vi "Timer On Delay.vi"(8 "error in":errorcluster, 10 "preset time (ms)":i32=1000, 11 "input":bool) -> (0 "error out":errorcluster, 2 "elapsed time (ms)":i32, 3 "output":bool)   [LabVIEW 2012, in "毫秒定时器.lvlib"]
uses:
  <vilib>/ptbypt/NI_PtbyPt.lvlib
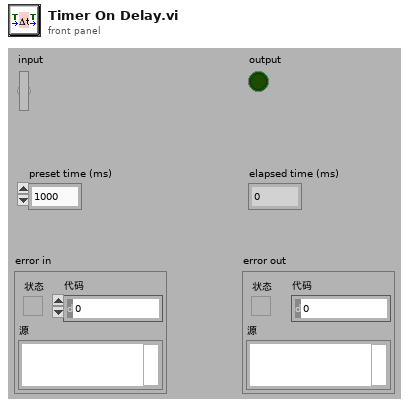
[diagram p1: front panel]
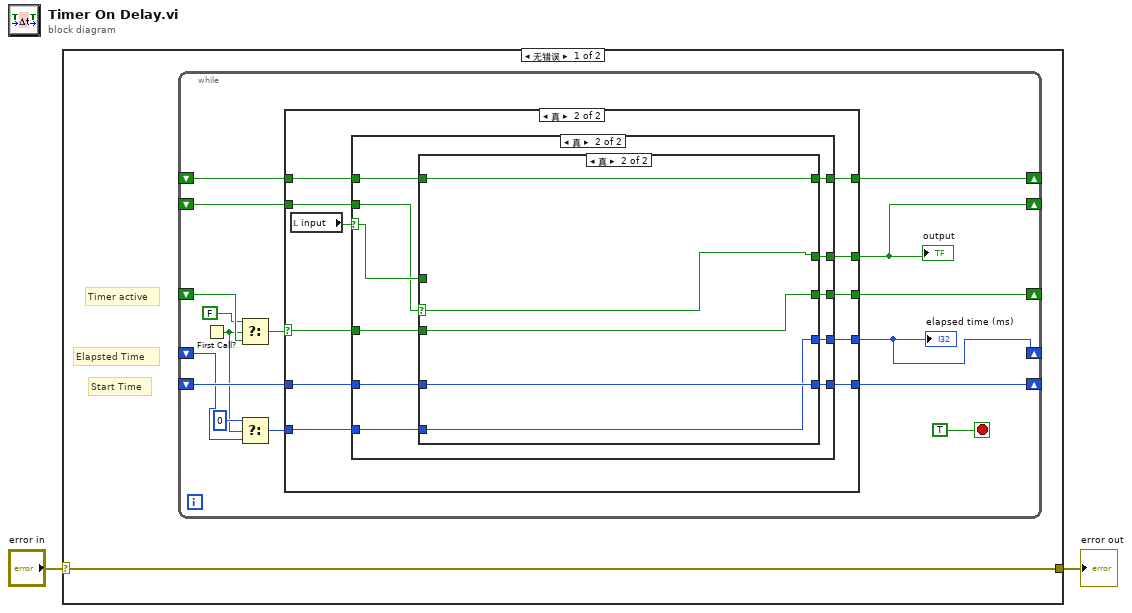
[diagram p0: block diagram]
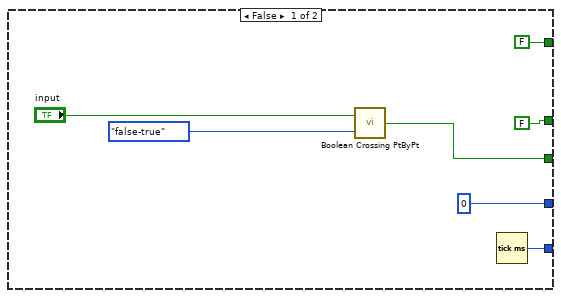
[diagram p2: hidden frame]
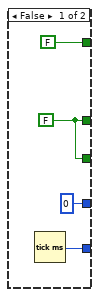
[diagram p3: hidden frame]
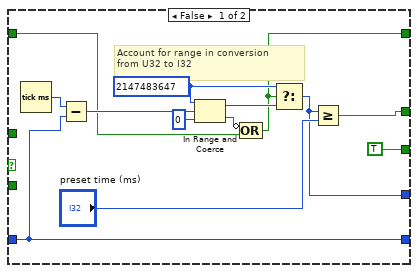
[diagram p4: hidden frame]
diagram:
  n1 = case shown="无错误" "error in" {
    selector: "error in" -> [w3 w71]
    tunnel: [w3 w71] -> w1
    frame No Error {
      # "Start Time"
      # "Elapsted Time"
      # "Timer active"
      n2 = while {
        shift-right: [w19] -> _
        shift-left: _ -> [w17]
        shift-right: [w16] -> _
        shift-left: _ -> [w15]
        shift-right: [w12] -> _
        shift-left: _ -> [w10]
        shift-right: [w8] -> _
        shift-left: _ -> [w6]
        shift-right: [w5] -> _
        shift-left: _ -> [w4]
        stop <- TRUE stop-if-true
        n3 = First Call?() -> (First Call?: T/F=w7:bool)
        n4 = Select(t=FALSE, s=w7, f=w15) -> (s? t:f=w13:bool)
        n5 = Select(t=u32 0 ("f"), s=w7, f=w10) -> (s? t:f=w9:u32)
        n6 = case shown="真" w13 {
          selector: w13 -> [_ w33]
          tunnel: [FALSE ("crossing") w37] -> w8
          tunnel: [u32 0 w36] -> w12
          tunnel: [w25 w30] -> w19
          tunnel: w17 -> [_ w31]
          tunnel: [w24 w32] -> w16
          tunnel: w9 -> [_ w34]
          tunnel: w6 -> [_ w29]
          tunnel: [FALSE w28] -> w5
          tunnel: w4 -> [_ w27]
          frame False {
            n7 = call <vilib>:"Boolean Crossing PtByPt.vi"("direction"=enum16{"either", "false-true", "true-false"}."false-true", "input"="input") -> ("crossing"=w24:bool)  [unwired: 1 in]
            n8 = Tick Count (ms)() -> (millisecond timer value=w25:u32)
          }
          frame True {
            n9 = local read "input"() -> (w35:bool)
            n10 = case shown="真" w35 {
              selector: w35 -> [_ w45]
              tunnel: w31 -> [_ w52]
              tunnel: [w40 w51] -> w37
              tunnel: [u32 0 ("f") w50] -> w36
              tunnel: [w40 w48] -> w32
              tunnel: w34 -> [_ w49]
              tunnel: w33 -> [_ w47]
              tunnel: [w39 w46] -> w30
              tunnel: w29 -> [_ w44]
              tunnel: [FALSE w43] -> w28
              tunnel: w27 -> [_ w42]
              frame False {
                w40 = FALSE
                n11 = Tick Count (ms)() -> (millisecond timer value=w39:u32)
              }
              frame True {
                n12 = case shown="真" w44 {
                  selector: w44 -> [_ w70]
                  tunnel: w52 -> [w61 w68]
                  tunnel: [w63 w70] -> w51
                  tunnel: [w56 w67] -> w50
                  tunnel: w49 -> [_ w67]
                  tunnel: [TRUE w69] -> w48
                  tunnel: w47 -> [_ w69]
                  tunnel: [w61 w68] -> w46
                  tunnel: w45 -> [_ _]
                  tunnel: [w54 w66] -> w43
                  tunnel: w42 -> [w53 w66]
                  frame False {
                    w60 = u32 2147483647 ("upper limit")
                    # "Account for range in conversion\nfrom U32 to I32"
                    n13 = Tick Count (ms)() -> (millisecond timer value=w65:u32)
                    n14 = Subtract(x=w65, y=w61) -> (x-y=w55:u32)
                    n15 = In Range and Coerce(upper limit=w60, x=w55, lower limit=u32 0) -> (coerced(x)=w59:u32, In Range?=w58:bool)
                    n16 = Compound Arithmetic op=OR(invert w58, w53) -> (w54:bool)
                    n17 = Select(t=w60, s=w54, f=w59) -> (s? t:f=w56:u32)
                    n18 = Greater Or Equal?(x=w56, y="preset time (ms)") -> (x >= y?=w63:bool)
                  }
                  frame True {
                  }
                }
              }
            }
          }
        }
        "output" <- w8
        "elapsed time (ms)" <- w12
      }
    }
    frame Error {
    }
  }
  "error out" <- w1
